vi "Comprar.vi"(8 "error in (no error)":errorcluster, 11 "Coca in":refnum<class "Coca.lvclass">) -> (0 "error out":errorcluster, 3 "Coca out":refnum<class "Coca.lvclass">)   [LabVIEW 2020, in "Coca.lvlib" / "Coca.lvclass"]
uses:
  Coca.lvclass
  C:/Program Files (x86)/National Instruments/LabVIEW 2020/vi.lib/ActorFramework/Actor/Actor.lvclass
  <vilib>/ActorFramework/Actor/Actor.lvclass/Actor.ctl
  Coca.lvclass/Coca.ctl
  UI Actor Messages/Buy Msg/Buy Msg.lvclass/Buy Msg.ctl
  <vilib>/ActorFramework/Message Enqueuer/Message Enqueuer.lvclass/Message Enqueuer.ctl
  <vilib>/ActorFramework/Message Enqueuer/Enqueue.vi
  UI Actor Messages/Buy Msg/Buy Msg.lvclass
  C:/Program Files (x86)/National Instruments/LabVIEW 2020/vi.lib/ActorFramework/Message/Message.lvclass
  <vilib>/ActorFramework/Message Priority Queue/Priority Enqueue.vi
  <vilib>/ActorFramework/Actor/Actor.lvclass
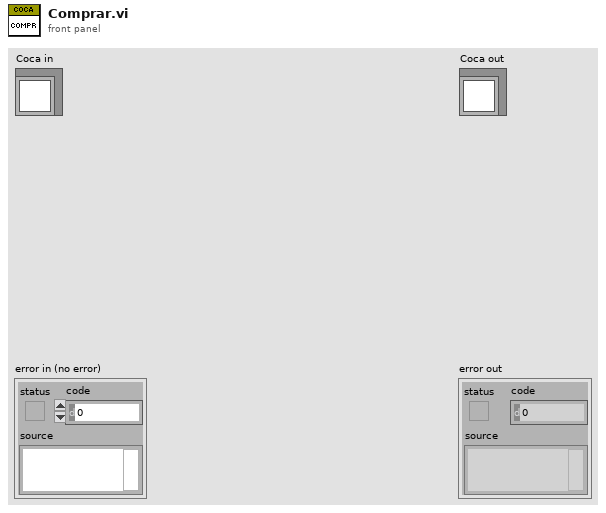
[diagram p1: front panel]
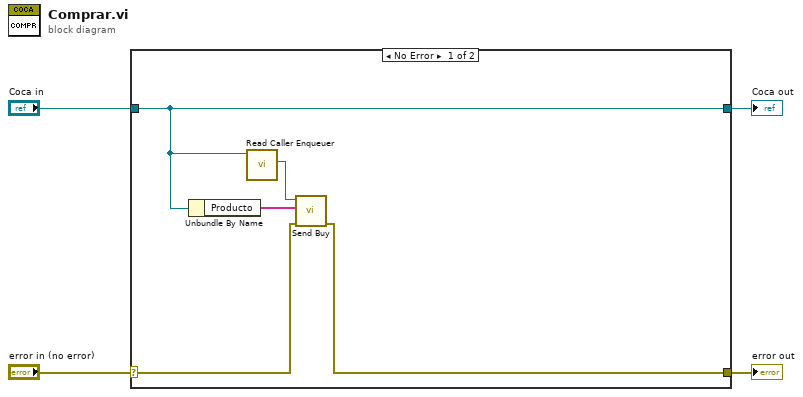
[diagram p0: block diagram]
diagram:
  n1 = case shown="No Error" "error in (no error)" {
    selector: "error in (no error)" -> [w6 w11]
    tunnel: [w5 w11] -> w3
    tunnel: [w9 w10] -> w1
    tunnel: "Coca in" -> [w9 w10]
    frame No Error {
      n2 = Unbundle By Name(w9) -> ("Producto"=w8:string[])
      n3 = call <vilib>:"Read Caller Enqueuer.vi"("Actor"=w9) -> ("Caller Enqueuer"=w7:refnum<class "Message Enqueuer.lvclass">)  [unwired: 10 in]
      n4 = call "Send Buy.vi"("error in (no error)"=w6, "Producto"=w8, "Message Enqueuer"=w7) -> ("error out"=w5:errorcluster)  [unwired: 7 in, 1 out]
    }
    frame Error {
    }
  }
  "error out" <- w3
  "Coca out" <- w1
